vi "gfitsio-write-history.vi"(8 "error in (no error)":errorcluster, 9 "history":string, 11 "gfits refnum":T1) -> (0 "error out":errorcluster, 3 "dup gfits refnum":T1)   [LabVIEW 2011, in "gfitsio.lvlib"]
doc: "Append a HISTORY keyword to the current HDU. The histroy string will be continued over multiple keywords if it is longer than 70 characters."
uses:
  gfitsio.lvlib
  gfitsio-refnum.ctl
  gfitsio.dll
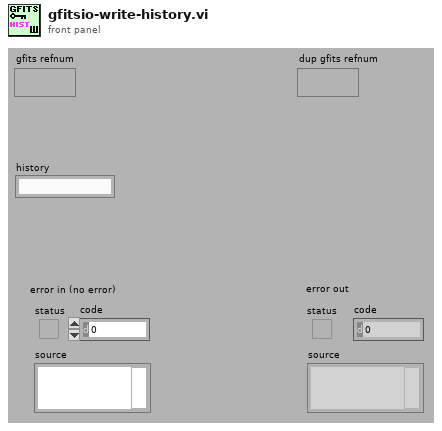
[diagram p1: front panel]
types:
  T1 = typedef "gfitsio.lvlib/gfitsio-refnum.ctl" = refnum<k1>
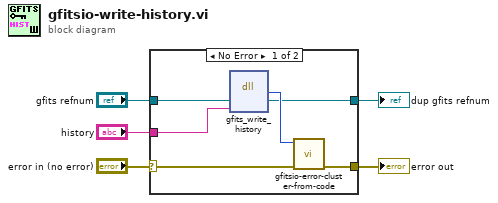
[diagram p0: block diagram]
diagram:
  n1 = case shown="No Error" "error in (no error)" {
    selector: "error in (no error)" -> [w10 w13]
    tunnel: [w9 w13] -> w2
    tunnel: "gfits refnum" -> [w6 w12]
    tunnel: [w7 w12] -> w4
    tunnel: "history" -> [w8 _]
    frame No Error {
      n2 = dll-call lib="C:/BonOMM/BonOMM-SAOMM/SubVIs/gfitsio/gfitsio.dll" fn="gfits_write_history"("gfits refnum"=w6, "history"=w8) -> (w11:i32, "gfits refnum"=w7:T1)  [unwired: 4 in, 2 out]
      n3 = call "gfitsio-error-cluster-from-code.vi"("error in (no error)"=w10, "error code"=w11) -> ("error out"=w9:errorcluster)  [unwired: 9 in]
    }
    frame Error {
    }
  }
  "error out" <- w2
  "dup gfits refnum" <- w4
